vi "Generate data for DIO FIFO.vi"(4 "Times, Ports, Lines, Values":i64[][](array[numeric])) -> (0 "Outputs of port C and D":u64[](array[numeric]), 1 "Outputs of port A and B":u64[](array[numeric]), 2 "Timing data":u64[](array[numeric]))   [LabVIEW 2017]
uses:
  globals/RIO and DAC defaults global.vi
  globals/DIO board parameters global.vi
panel:
  out "prev":i32[](array[numeric])=[-32634, 69]
  out "all times":i64[](array[numeric])=[0, 0, 0, 0, 0, 1000, 1000, 3000, 3000, 3000]
  out "all values":i32[](array[numeric])=[1, 1, 1, 0, 0, 0, 1, 1, 1, 0]
  out "all ports":i32[](array[numeric])=[0, 0, 0, 1, 1, 0, 1, 0, 1, 1]
  out "all lines":i32[](array[numeric])=[1, 2, 2, 1, 1, 2, 15, 2, 0, 15]
  # "time (2 words)  port0      1           2       3"
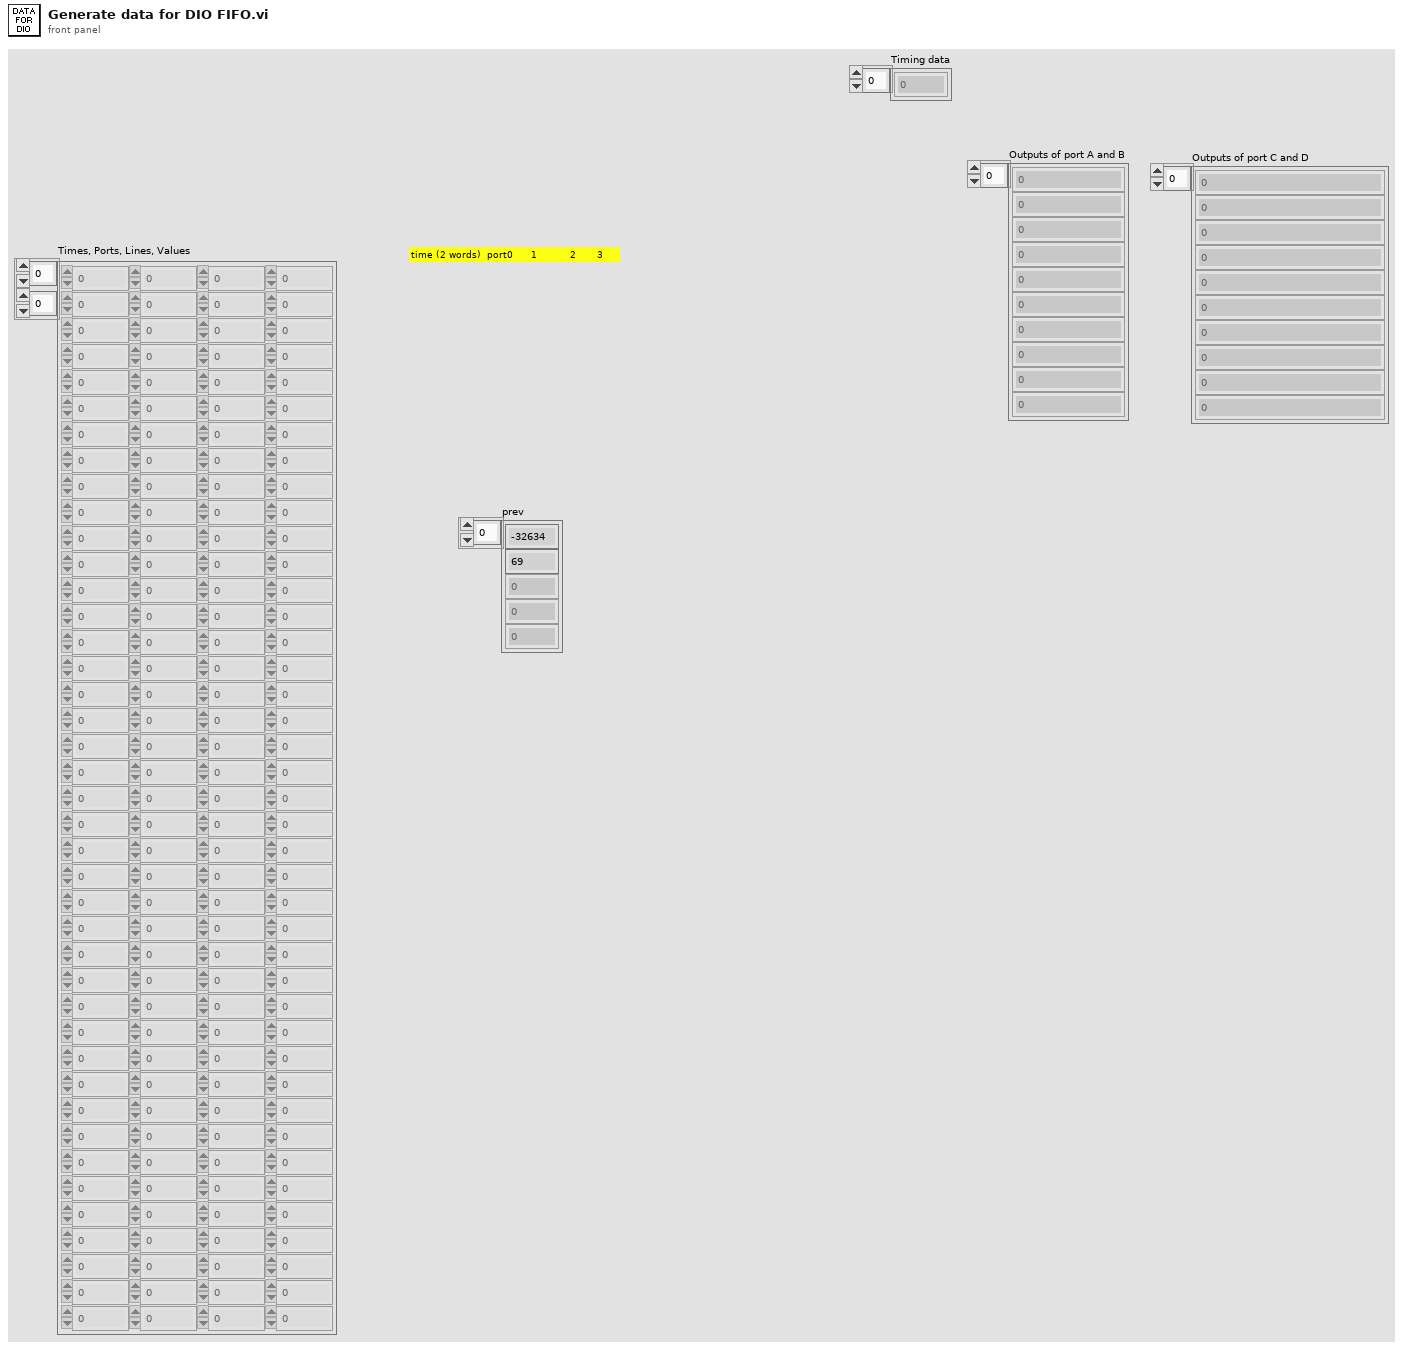
[diagram p1: front panel]
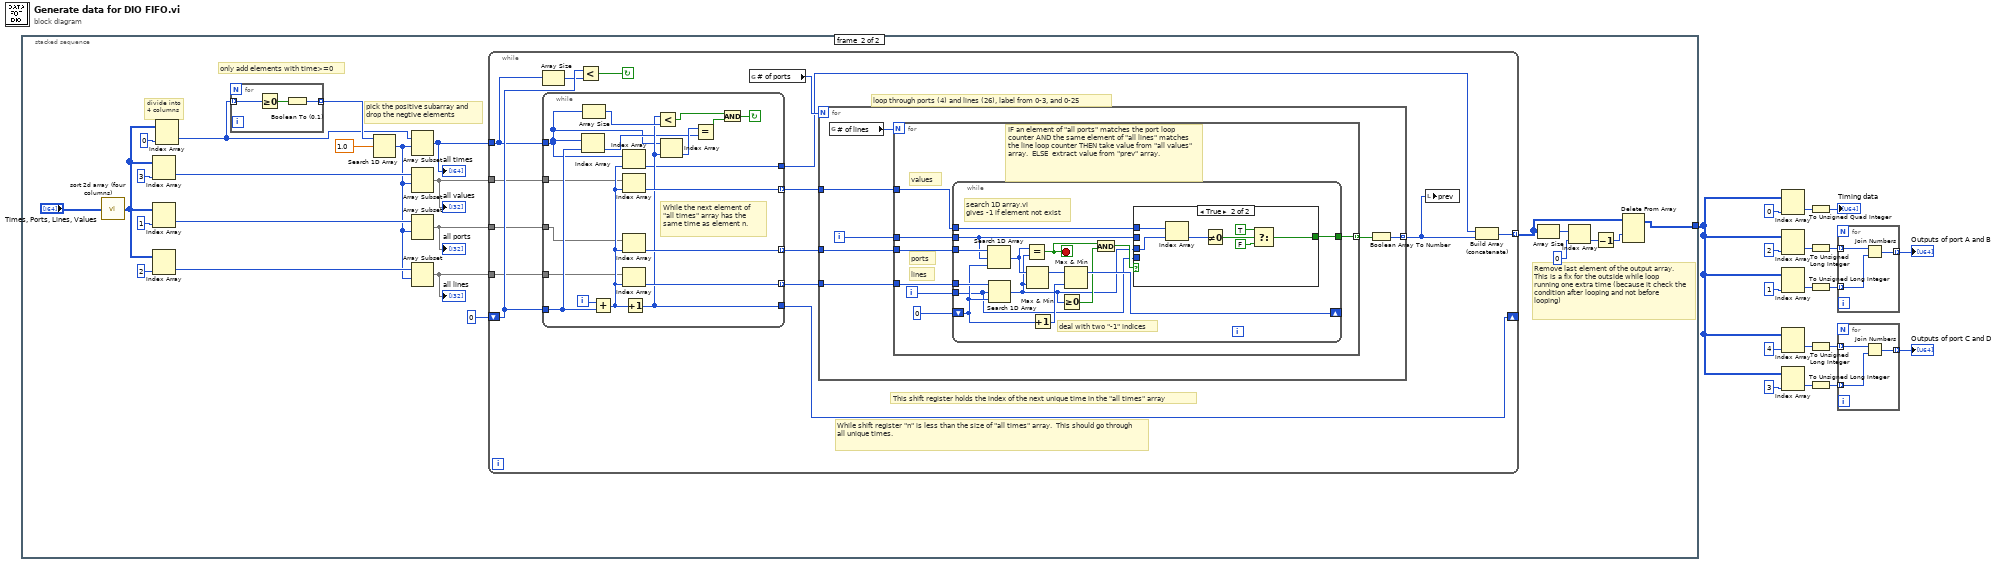
[diagram p0: block diagram]
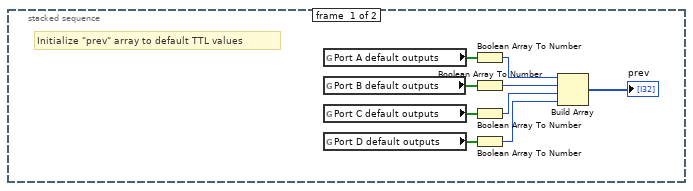
[diagram p2: hidden frame]
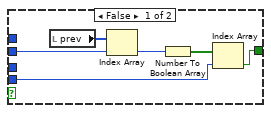
[diagram p3: hidden frame]
diagram:
  n1 = stacked-sequence {
    tunnel: [_ w28] -> w17
    frame #0 {
      # "Initialize \"prev\" array to default TTL values"
      n2 = global read "RIO and DAC defaults global.vi" "Port A default outputs"() -> (w27:bool[])
      n3 = global read "RIO and DAC defaults global.vi" "Port B default outputs"() -> (w26:bool[])
      n4 = global read "RIO and DAC defaults global.vi" "Port C default outputs"() -> (w25:bool[])
      n5 = global read "RIO and DAC defaults global.vi" "Port D default outputs"() -> (w24:bool[])
      n6 = Boolean Array To Number(Boolean array=w27) -> (number=w23:i32)
      n7 = Boolean Array To Number(Boolean array=w26) -> (number=w22:i32)
      n8 = Boolean Array To Number(Boolean array=w25) -> (number=w21:i32)
      n9 = Boolean Array To Number(Boolean array=w24) -> (number=w20:i32)
      n10 = Build Array(w23, w22, w21, w20) -> (→"prev":i32[])
    }
    frame #1 {
      # "pick the positive subarray and \ndrop the negtive elements"
      # "Remove last element of the output array. This is a fix for the outside while loop running one extra time (because it check the condition after looping and not before looping)"
      # "divide into 4 columns"
      # "only add elements with time>=0"
      n11 = call "sort 2d array (four columns).vi"("2D array to sort"="Times, Ports, Lines, Values") -> ("Sorted array"=w51:i64[][])
      n12 = Index Array(array=w51, index (col)=i8 3 ("Column #")) -> (element=w32:i64[])  [unwired: 1 in]
      n13 = Index Array(array=w51, index (col)=i8 1 ("Column #")) -> (element=w30:i64[])  [unwired: 1 in]
      n14 = Index Array(array=w51, index (col)=i8 2 ("Column #")) -> (element=w31:i64[])  [unwired: 1 in]
      n15 = Index Array(array=w51, index (col)=i8 0 ("Column #")) -> (element=w37:i64[])  [unwired: 1 in]
      n16 = for {
        tunnel: w37 -> [w129] mode=indexing
        tunnel: [w127] -> w50 mode=indexing
        n17 = Greater Or Equal To 0?(x=w129) -> (x >= 0?=w128:bool)
        n18 = Boolean To (0,1)(Boolean=w128) -> (0, 1=w127:i16)
      }
      n19 = Search 1D Array(1D array=w50, element=1.0) -> (index of element=w29:i32)  [unwired: 1 in]
      n20 = Array Subset(array=w37, index=w29) -> (w36:i64[])  [unwired: 1 in]
      "all times" <- w36
      n21 = Array Subset(array=w32, index=w29) -> (w33:i64[])  [unwired: 1 in]
      "all values" <- w33
      n22 = Array Subset(array=w30, index=w29) -> (w35:i64[])  [unwired: 1 in]
      "all ports" <- w35
      n23 = Array Subset(array=w31, index=w29) -> (w34:i64[])  [unwired: 1 in]
      "all lines" <- w34
      n24 = while {
        tunnel: w35 -> [w55]
        tunnel: w34 -> [w56]
        tunnel: w33 -> [w57]
        tunnel: w36 -> [w54]
        tunnel: [w66] -> w43 mode=indexing
        shift-left: 0 -> [w59]
        shift-right: [w60] -> _
        stop <- w65 continue-if-true
        # "loop through ports (4) and lines (26), label from 0-3, and 0-25"
        # "This shift register holds the index of the next unique time in the \"all times\" array"
        # "While shift register \"n\" is less than the size of \"all times\" array.  This should go through all unique times."
        n25 = Array Size(array=w54) -> (size(s)=w58:i32)
        n26 = while {
          tunnel: w55 -> [w70]
          tunnel: w56 -> [w71]
          tunnel: w57 -> [w72]
          tunnel: w54 -> [w69]
          tunnel: [w73] -> w53
          tunnel: w59 -> [w76]
          tunnel: [w77] -> w60
          tunnel: [w82] -> w61 mode=indexing
          tunnel: [w83] -> w62 mode=indexing
          tunnel: [w84] -> w63 mode=indexing
          i -> [w79]
          stop <- w80 continue-if-true
          # "While the next element of \"all times\" array has the same time as element n."
          n27 = Index Array(array=w69, index=w76) -> (element=w74:i64)
          n28 = Array Size(array=w69) -> (size(s)=w81:i32)
          n29 = Add(x=w79, y=w76) -> (x+y=w78:i32)
          n30 = Index Array(array=w69, index=w78) -> (element=w73:i64)
          n31 = Index Array(array=w72, index=w78) -> (element=w82:i64)
          n32 = Index Array(array=w70, index=w78) -> (element=w84:i64)
          n33 = Index Array(array=w71, index=w78) -> (element=w83:i64)
          n34 = Increment(x=w78) -> (x+1=w77:i32)
          n35 = Less?(x=w77, y=w81) -> (x < y?=w68:bool)
          n36 = Index Array(array=w69, index=w77) -> (element=w75:i64)
          n37 = Equal?(x=w75, y=w74) -> (x = y?=w67:bool)
          n38 = And(x=w68, y=w67) -> (x .and. y?=w80:bool)
        }
        n39 = Less?(x=w59, y=w58) -> (x < y?=w65:bool)
        n40 = global read "DIO board parameters global.vi" "# of ports"() -> (w64:u16)
        n41 = for {
          N: w64 -> [_]
          tunnel: w63 -> [w90]
          tunnel: w62 -> [w89]
          tunnel: w61 -> [w88]
          tunnel: [w87] -> w52 mode=indexing
          i -> [w91]
          n42 = global read "DIO board parameters global.vi" "# of lines"() -> (w85:u16)
          n43 = for {
            N: w85 -> [_]
            tunnel: w91 -> [w97]
            tunnel: w90 -> [w98]
            tunnel: w89 -> [w96]
            tunnel: w88 -> [w94]
            tunnel: [w92] -> w86 mode=indexing
            i -> [w95]
            # "lines"
            # "ports"
            # "values"
            # "IF an element of \"all ports\" matches the port loop counter AND the same element of \"all lines\" matches the line loop counter THEN take value from \"all values\" array.  ELSE  extract value from \"prev\" array."
            n44 = while {
              tunnel: [w107] -> w92
              tunnel: w94 -> [w111]
              tunnel: w96 -> [w112]
              tunnel: w97 -> [w100]
              tunnel: w98 -> [w113]
              tunnel: w95 -> [w99]
              shift-left: 0 -> [w110]
              shift-right: [w108] -> _
              stop <- w104 stop-if-true
              # "deal with two \"-1\" indices"
              # "search 1D array.vi\ngives -1 if element not exist"
              n45 = Search 1D Array(1D array=w113, element=w100, start index (0)=w110) -> (index of element=w102:i32)
              n46 = Search 1D Array(1D array=w112, element=w99, start index (0)=w110) -> (index of element=w101:i32)
              n47 = Equal?(x=w102, y=w101) -> (x = y?=w104:bool)
              n48 = Max & Min(x=w102, y=w101) -> (max(x,y)=w105:i32)  [unwired: 1 out]
              n49 = Increment(x=w110) -> (x+1=w109:i32)
              n50 = Greater Or Equal To 0?(x=w101) -> (x >= 0?=w103:bool)
              n51 = Max & Min(x=w105, y=w109) -> (max(x,y)=w108:i32)  [unwired: 1 out]
              n52 = And(x=w104, y=w103) -> (x .and. y?=w106:bool)
              n53 = case shown="True" w106 {
                tunnel: w101 -> [_ w126]
                tunnel: w111 -> [_ w125]
                tunnel: w100 -> [w116 _]
                tunnel: [w115 w122] -> w107
                tunnel: w99 -> [w114 _]
                frame False {
                  n54 = local read "prev"() -> (w117:i32[])
                  n55 = Index Array(array=w117, index=w116) -> (element=w118:i32)
                  n56 = Number To Boolean Array(number=w118) -> (Boolean array=w119:bool[])
                  n57 = Index Array(array=w119, index=w114) -> (element=w115:bool)
                }
                frame True {
                  n58 = Index Array(array=w125, index=w126) -> (element=w120:i64)
                  n59 = Not Equal To 0?(x=w120) -> (x != 0?=w123:bool)
                  n60 = Select(t=TRUE, s=w123, f=FALSE) -> (s? t:f=w122:bool)
                }
              }
            }
          }
          n61 = Boolean Array To Number(Boolean array=w86) -> (number=w87:i32)
        }
        n62 = local write "prev"(w52) -> ()
        n63 = Build Array (concatenate)(w53, w52) -> (w66:i64[])
      }
      n64 = Array Size(array=w43) -> (size(s)=w42:i32[])
      n65 = Index Array(array=w42, index=0 ("Index")) -> (element=w41:i32)
      n66 = Decrement(x=w41) -> (x-1=w40:i32)
      n67 = Delete From Array(array=w43, index (row)=w40) -> (array with subset deleted=w28:i64[][])  [unwired: 2 in, 1 out]
    }
  }
  n68 = Index Array(array=w17, index (col)=0 ("disabled index (col)")) -> (element=w2:i64[])  [unwired: 1 in]
  n69 = Index Array(array=w17, index (col)=2 ("disabled index (col)")) -> (element=w11:i64[])  [unwired: 1 in]
  n70 = Index Array(array=w17, index (col)=1 ("disabled index (col)")) -> (element=w12:i64[])  [unwired: 1 in]
  n71 = Index Array(array=w17, index (col)=4 ("disabled index (col)")) -> (element=w6:i64[])  [unwired: 1 in]
  n72 = Index Array(array=w17, index (col)=3 ("disabled index (col)")) -> (element=w7:i64[])  [unwired: 1 in]
  n73 = To Unsigned Quad Integer(1:w2) -> (0:→"Timing data":u64[])
  n74 = To Unsigned Long Integer(number=w11) -> (unsigned 32bit integer=w9:u32[])
  n75 = To Unsigned Long Integer(number=w12) -> (unsigned 32bit integer=w10:u32[])
  n76 = To Unsigned Long Integer(number=w6) -> (unsigned 32bit integer=w4:u32[])
  n77 = To Unsigned Long Integer(number=w7) -> (unsigned 32bit integer=w3:u32[])
  n78 = for {
    tunnel: w10 -> [w132] mode=indexing
    tunnel: w9 -> [w131] mode=indexing
    tunnel: [w130] -> w8 mode=indexing
    n79 = Join Numbers(hi=w131, lo=w132) -> ((hi.lo)=w130:u64)
  }
  "Outputs of port A and B" <- w8
  n80 = for {
    tunnel: w3 -> [w135] mode=indexing
    tunnel: w4 -> [w134] mode=indexing
    tunnel: [w133] -> w5 mode=indexing
    n81 = Join Numbers(hi=w134, lo=w135) -> ((hi.lo)=w133:u64)
  }
  "Outputs of port C and D" <- w5
